vi "G4SubTemplate_Singleton_5x6x5_ReadWriteAttribute.vi"(11 "error in (no error)":errorcluster) -> (15 "error out":errorcluster)   [LabVIEW 2020]
uses:
  <resource>/Framework/Providers/Open_GDS/ClassProviders/Provider_EndevoGOOP400/Templates/G4SubTemplate_Singleton_5x6x5/G4SubTemplate_Singleton_5x6x5.lvclass
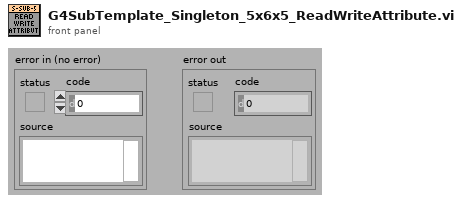
[diagram p1: front panel]
types:
  T1 = typedef "G4SubTemplate_Singleton_5x6x5.lvclass/ObjectAttributes.ctl" = cluster{"Attribute1":dbl}
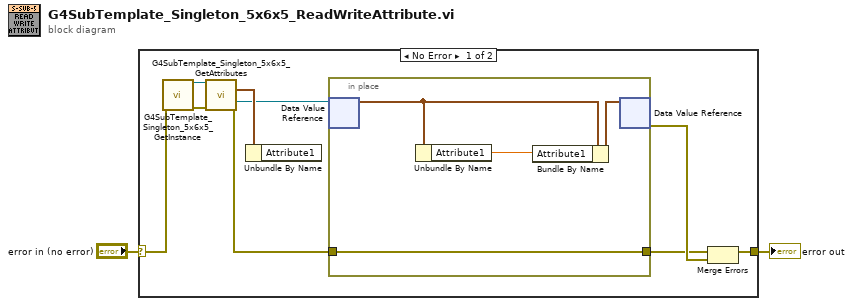
[diagram p0: block diagram]
diagram:
  n1 = case shown="No Error" "error in (no error)" {
    selector: "error in (no error)" -> [w6 w16]
    tunnel: [w9 w16] -> w1
    frame No Error {
      n2 = call <resource>:"G4SubTemplate_Singleton_5x6x5_GetInstance.vi"("error in (no error)"=w6) -> ("reference out"=w7:refnum<class "G4SubTemplate_Singleton_5x6x5.lvclass">, "error out"=w8:errorcluster)  [unwired: 10 in, 3 out]
      n3 = call <resource>:"G4SubTemplate_Singleton_5x6x5_GetAttributes.vi"("reference in"=w7, "error in (no error)"=w8) -> ("Data"=w11:T1, "DataRef"=w5:refnum<data-value>, "error out"=w4:errorcluster)  [unwired: 10 in, 1 out]
      n4 = Unbundle By Name(w11) -> ()  [unwired: 1 out]
      n5 = in-place {
        in-place-border: w4 -> [w14]
        in-place-border: [w14] -> w3
        n6 = in-place-dvr #1(w5) -> (w13:T1)  [unwired: 1 out]
        n7 = Unbundle By Name(w13) -> ("Attribute1"=w12:dbl)
        n8 = Bundle By Name(cluster=w13, "Attribute1"=w12) -> (w15:T1)
        n9 = in-place-dvr #1(w15) -> (w10:errorcluster)  [unwired: 1 out]
      }
      n10 = Merge Errors(w3, w10) -> (w9:errorcluster)
    }
    frame Error {
    }
  }
  "error out" <- w1
